vi "HRTF Measurement.vi"(9 "Device Config":T4={"TDT"={"Output"={"Device"=enum."RZ5", "Num"=0}, "Input"=enum."Front Panel"}, "Transducer"="", "Properties"={"Amplifier"=enum."None", "Panic button"=FALSE}, "System"=enum."PXI"}) -> ()   [LabVIEW 2015]
uses:
  EPhys/LV Source/Typedefs/EPhys-Hardware Config.ctl
  PXI DAQ VIs/TDT VIs/Typedefs/TDT-Device Config.ctl
  PXI DAQ VIs/TDT VIs/Typedefs/TDT-Output source.ctl
  PXI DAQ VIs/TDT VIs/Typedefs/TDT-Device ID.ctl
  PXI DAQ VIs/TDT VIs/Typedefs/TDT-Input source.ctl
  EPhys/LV Source/Typedefs/EPhys-Hardware Properties.ctl
  PXI DAQ VIs/Type Defs/Hardware Destination.ctl
  Typedefs/HRTF Config/HRTF Config.xctl
  Utility VIs/Buttons/KCheckmarkBoolean 2.ctl
  Typedefs/HRTF-Result.ctl
  Typedefs/HRTF-Parameters.ctl
  Typedefs/HRTF-Waveform.ctl
  Typedefs/HRTF-Window.ctl
  Typedefs/HRTF-Window Type.ctl
  Typedefs/HRTF-State.ctl
  Typedefs/HRTF-Options.ctl
  Typedefs/HRTF-Hardware Config (TDT).ctl
  Typedefs/HRTF-State Machine Action.ctl
  Typedefs/HRTF-Runtime Data.ctl
  <vilib>/Analysis/2dsp.llb/Real FFT.vi
  <vilib>/Utility/miscctls.llb/LVBoundsTypeDef.ctl
  <vilib>/Analysis/NI_AALPro.lvlib
panel:
  in  "Compute":bool
  in  "Window":T1={"Window"=0, "Length (ms)"=50.0, "Center (ms)"=50.0} {"Window" items=["None", "Rectangle", "Hanning"]}
  in  "Cancel":bool
  in  "Apply":bool
  out "Result":T2
  out "StimDur":dbl format="%#_3g ms"
  in  "wftab":enum32{"Page 1", "Page 2"}(tab)
  in  "Freq Step (Hz)":dbl=50.0
  in  "Seed":i32=50
  in  "Order":i32=50
  in  "Attenuation (dB)":dbl=30.0
  in  "Sample Rate (Hz)":dbl=100000.0
  in  "Waveform":enum16{"Chirp", "MLS"}(ring)
  out "Progress":u8(slide) scale=0.0..1.0
  in  "Elevation":u16(ring) items=["0°", "7.5°", "15°", "22.5°", "30°", "37.5°", "45°", "52.5°", "60°", "67.5°", "75°", "82.5°", "90°", "97.5°", "105°", "112.5°", "120°", "127.5°", "135°", "142.5°", "150°", "157.5°", "165°", "172.5°", "180°"]
  in  "Speaker only":T3
  in  "Start":bool
  in  "Stop":bool
  in  "Subject ID":string
  in  "Config":i32(xcontrol)
  in  "Averages":i32=128
  in  "Data Tab":enum32{"Stimulus", "Response", "HRTFs"}(tab)
  out "StimPhase":cluster{i32, "dx":dbl, "Y":dbl[]}(graph)
  out "StimMag":cluster{i32, "dx":dbl, "Y":dbl[]}(graph)
  out "StimAutocorr":cluster{dbl, "dx":dbl, "Y":dbl[]}(graph) caption="Autocorrelation"
  out "Stimulus (time)":cluster{i32, "dx":dbl, "Y":dbl[]}(graph) caption="Amplitude"
  out "RespTime":cluster{"offset":dbl, "dx":dbl, "Y":dbl[][]}(graph) caption="Amplitude"
  in  "RespFiles":u16(ring) items=["", "Speaker-elev0-az-90", "Speaker-elev0-az-82.5", "Speaker-elev0-az-75", "Speaker-elev0-az-67.5", "Speaker-elev0-az-60", "Speaker-elev0-az-52.5", "Speaker-elev0-az-45"]
  out "RespCorr":cluster{"offset":dbl, "dx":dbl, "Y":dbl[][]}(graph) caption="Impulse Response"
  out "RespMag":cluster{"offset":dbl, "dx":dbl, "Y":dbl[][]}(graph)
  out "RespPhase":cluster{"offset":dbl, "dx":dbl, "Y":dbl[][]}(graph)
  out "Status":string
  in  "HRTFFiles":u16(ring) items=["", "HRTF-elev0-az-90", "HRTF-elev0-az-82.5", "HRTF-elev0-az-75", "HRTF-elev0-az-67.5", "HRTF-elev0-az-60", "HRTF-elev0-az-52.5", "HRTF-elev0-az-45", "HRTF-elev0-az-37.5", "HRTF-elev0-az-30", "HRTF-elev0-az-22.5", "HRTF-elev0-az-15", "HRTF-elev0-az-7.5", "HRTF-elev0-az0", "HRTF-elev0-az7.5", "HRTF-elev0-az15", "HRTF-elev0-az22.5", "HRTF-elev0-az30", "HRTF-elev0-az37.5", "HRTF-elev0-az45", "HRTF-elev0-az52.5", "HRTF-elev0-az60", "HRTF-elev0-az67.5", "HRTF-elev0-az75", "HRTF-elev0-az82.5", "HRTF-elev0-az90"]
  out "HRTFMag":cluster{"offset":dbl, "dx":dbl, "Y":dbl[][]}(graph)
  out "HRTFPhase":cluster{"offset":dbl, "dx":dbl, "Y":dbl[][]}(graph)
  out "HRIR":cluster{"offset":dbl, "dx":dbl, "Y":dbl[][]}(graph) caption="Impulse Response"
  # "Stimulus"
  # "HRTF"
  # "Response"
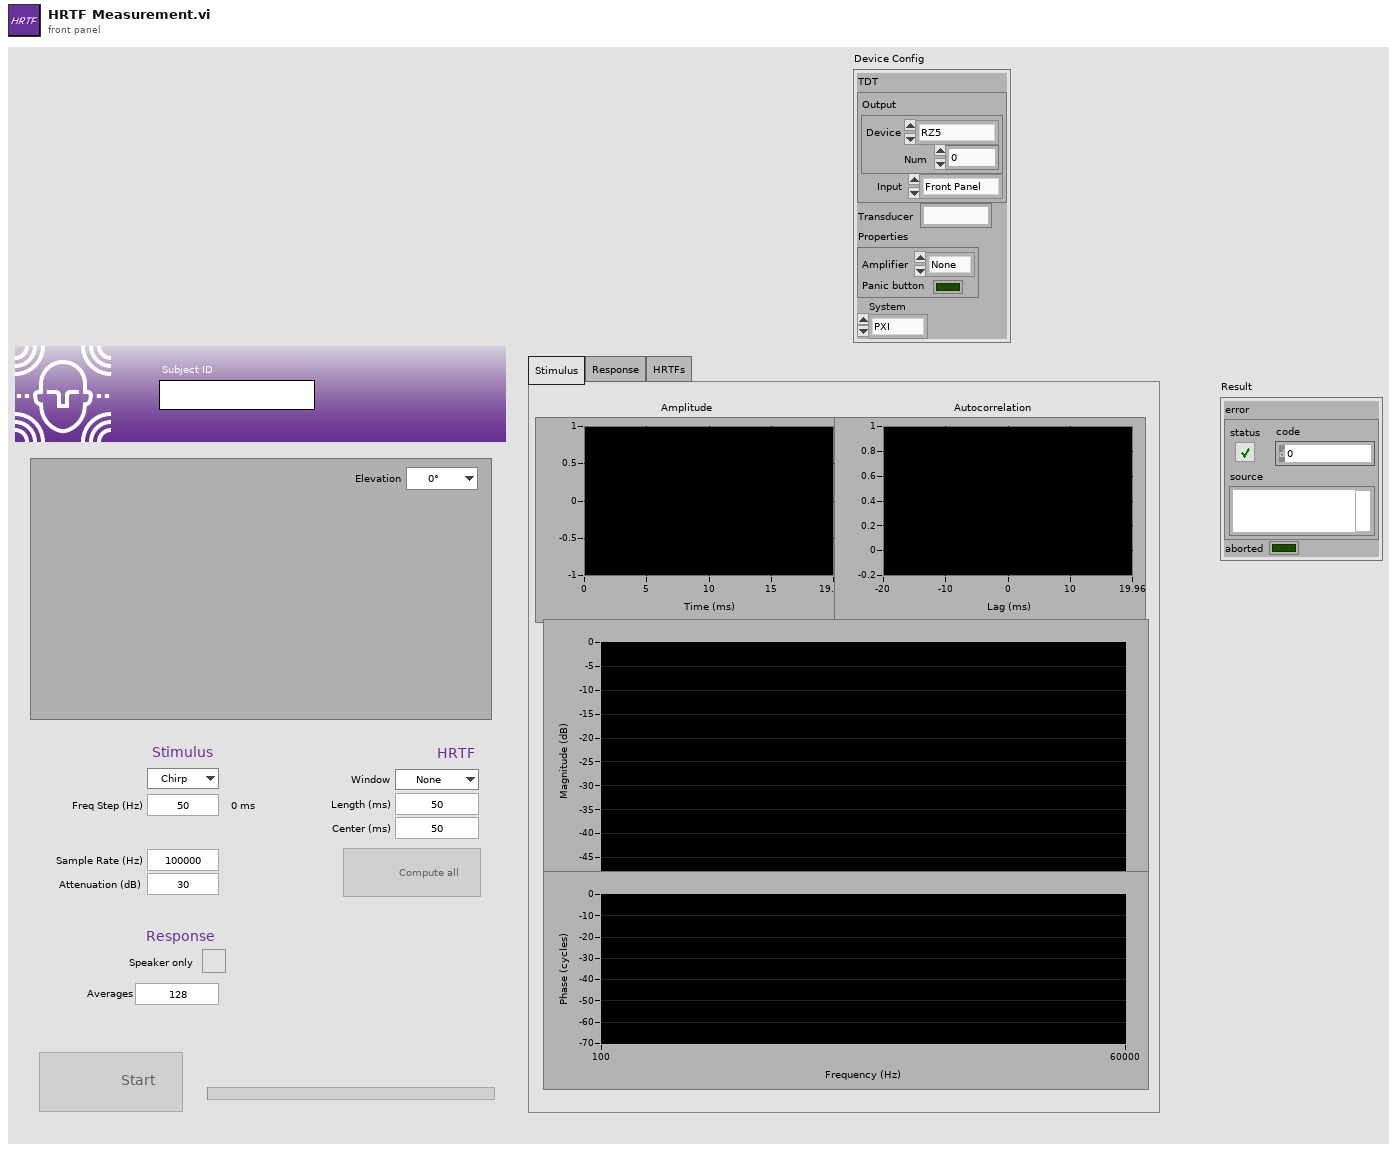
[diagram p1: front panel]
types:
  T1 = cluster{"Window":u16, "Length (ms)":dbl, "Center (ms)":dbl}
  T2 = typedef "HRTF-Result.ctl" = cluster{"error":errorcluster, "aborted":bool}
  T3 = typedef "KCheckmarkBoolean 2.ctl" = bool
  T4 = typedef "EPhys-Hardware Config.ctl" = cluster{"TDT":T5, "Transducer":string, "Properties":T9, "System":T10}
  T5 = typedef "TDT-Device Config.ctl" = cluster{"Output":T6, "Input":T8}
  T6 = typedef "TDT-Output source.ctl" = cluster{"Device":T7, "Num":i32}
  T7 = typedef "TDT-Device ID.ctl" = enum16{"None", "PA5", "RP2", "RL2", "RA16", "RV8", "RX5", "RX6", "RX7", "RX8", "RZ2", "RZ5", "RZ6"}
  T8 = typedef "TDT-Input source.ctl" = enum16{"Front Panel", "RA4LI", "RA16LI"}
  T9 = typedef "EPhys-Hardware Properties.ctl" = cluster{"Amplifier":enum16{"None", "Biosemi", "Eclipse", "Eclipse (N.C.)", "Grass"}, "Panic button":bool}
  T10 = typedef "Hardware Destination.ctl" = enum16{"None", "PXI", "TDT", "NI", "TDTSIM"}
  T11 = typedef "HRTF-Parameters.ctl" = cluster{"Fs (Hz)":dbl, "atten (dB)":dbl, "Waveform":T12, "Freq Res (Hz)":dbl, "Order":i32, "Averages":i32, "seed":i64, "Window":T13}
  T12 = typedef "HRTF-Waveform.ctl" = enum16{"Chirp", "MLS"}
  T13 = typedef "HRTF-Window.ctl" = cluster{"Type":T14, "Length (ms)":dbl, "Center (ms)":dbl}
  T14 = typedef "HRTF-Window Type.ctl" = enum16{"None", "Rectangle", "Hanning"}
  T15 = typedef "HRTF-Options.ctl" = cluster{"Root folder":path, "Elevations":string, "Wait (s)":dbl, "Azimuths":dbl[]}
  T16 = typedef "HRTF-State.ctl" = cluster{"Folder":path, "Elevation":dbl, "iAzimuth":i32, "Mic":i32, "speaker only":bool, "ID":string, "Azimuth":dbl}
  T17 = typedef "LVBoundsTypeDef.ctl" = cluster{"Width":u32, "Height":u32}
  T18 = cluster{"Options":T15, "Params":T11, "State":T16}
  T19 = enum8{"Enabled", "Disabled", "Disabled and Grayed Out"}
  T20 = enum32{"Invalid", "Standard", "Closed", "Hidden", "Minimized", "Maximized"}
  T21 = typedef "LVRangeTypeDef.ctl" = cluster{"Minimum":dbl, "Maximum":dbl, "Increment":dbl, "Minor Increment":dbl, "Start":dbl}
  T22 = typedef "HRTF-Hardware Config (TDT).ctl" = cluster{"Output":T6, "Speaker":cluster{"Channel":i32, "Primary mux":i32, "Secondary mux":i32}, "Right mic":i32, "Left mic":i32}
  T23 = typedef "HRTF-Runtime Data.ctl" = cluster{"StimSpec":cdb[][], "Mic Sum":dbl[][], "df (Hz)":dbl, "dt (ms)":dbl, "Navg":i32, "Nacq":i32, "pts/rep":i32, "reps/frame":i32, "Stimulus":dbl[]}
  T24 = typedef "HRTF-State Machine Action.ctl" = enum16{"Wait", "Init", "Multiplex", "Measure", "Save", "End"}
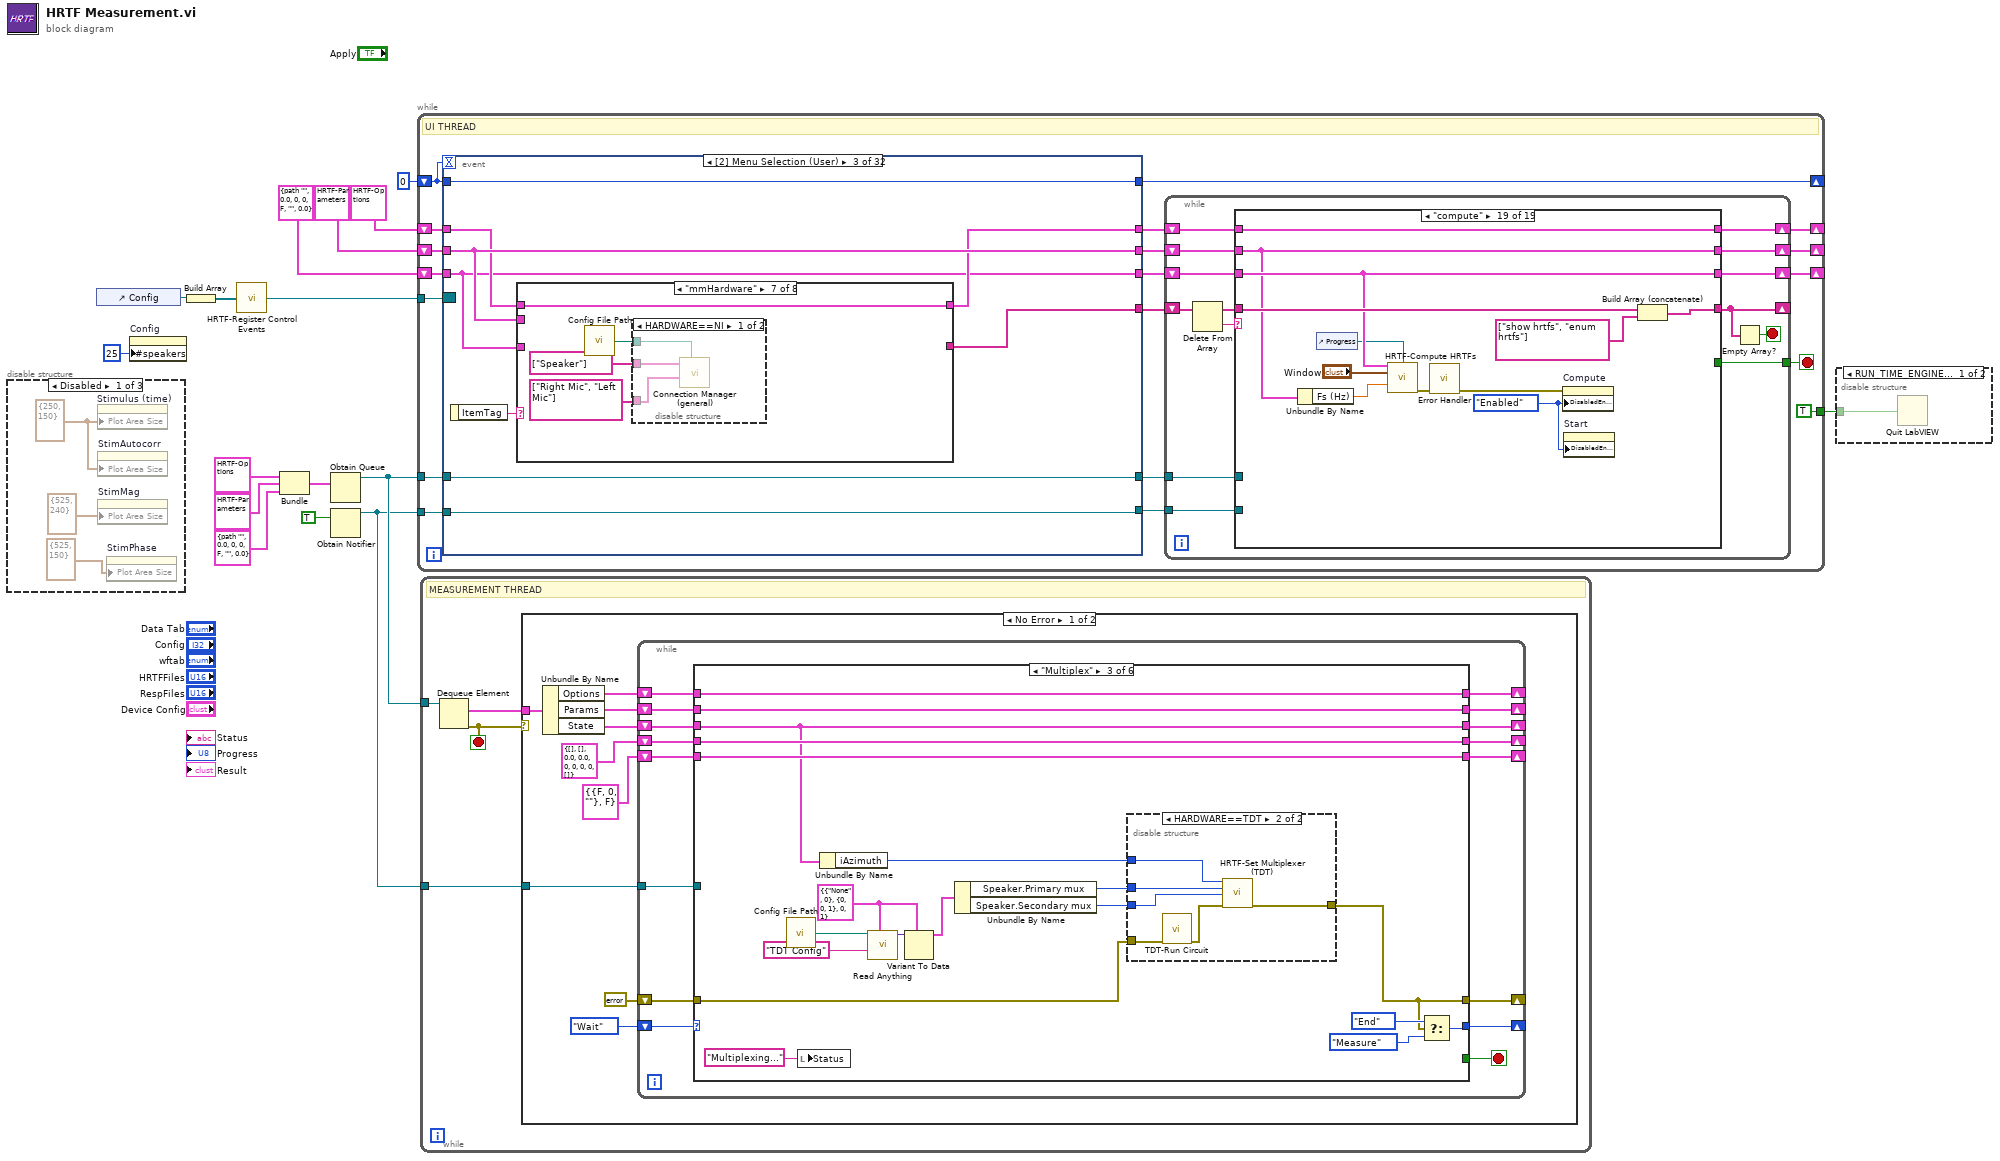
[diagram p0: block diagram]
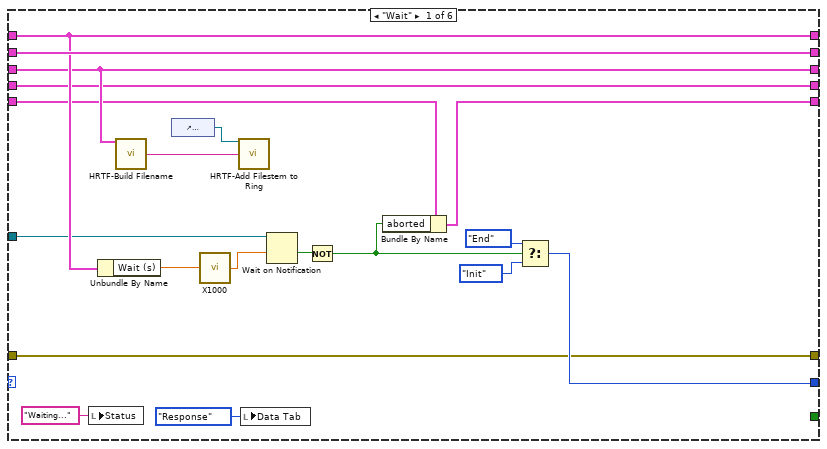
[diagram p2: hidden frame]
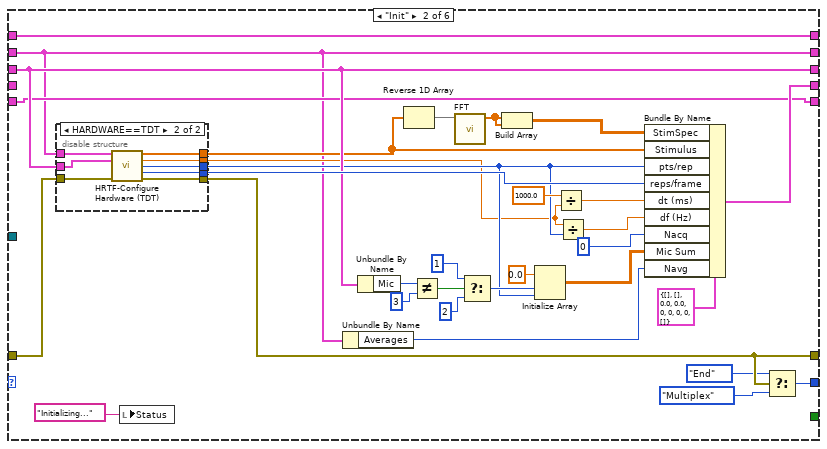
[diagram p3: hidden frame]
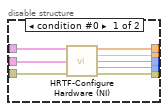
[diagram p4: hidden frame]
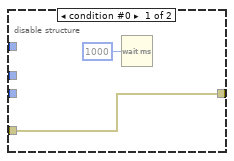
[diagram p5: hidden frame]
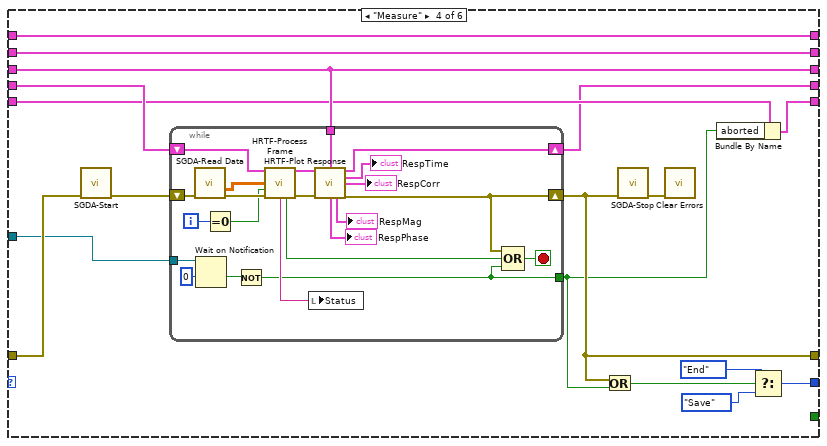
[diagram p6: hidden frame]
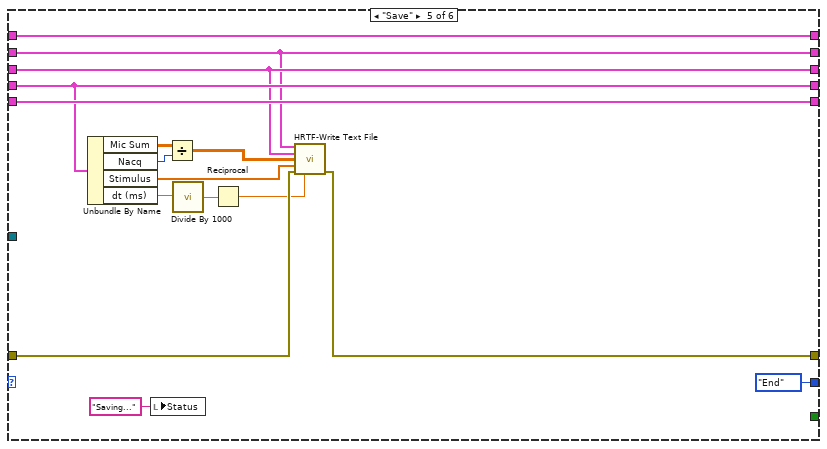
[diagram p7: hidden frame]
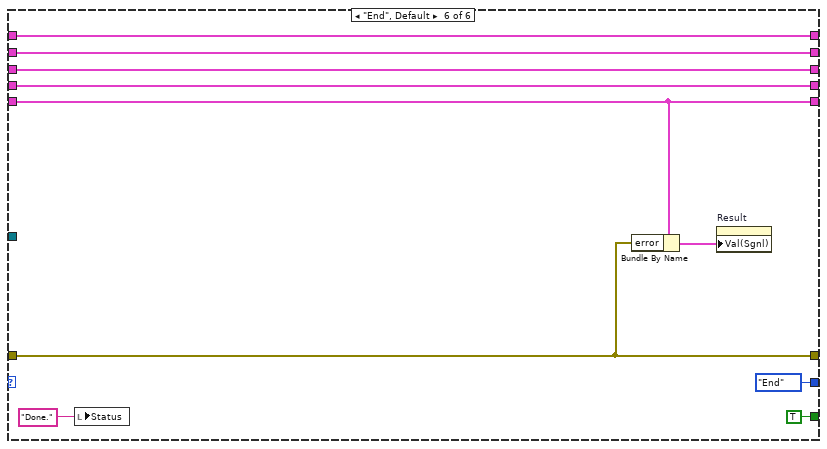
[diagram p8: hidden frame]
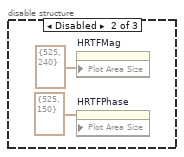
[diagram p10: hidden frame]
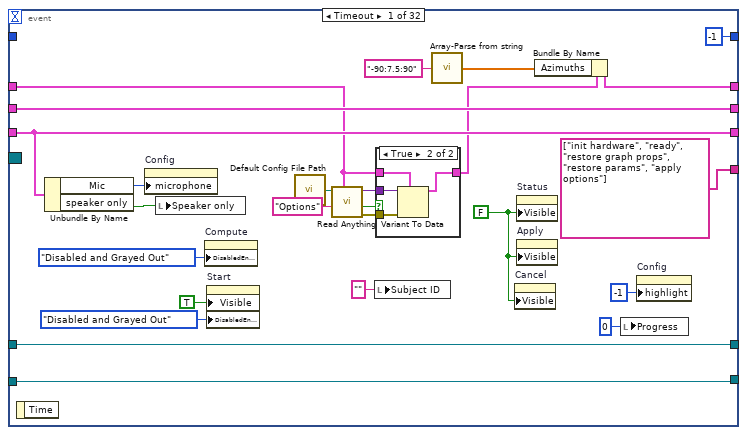
[diagram p12: hidden frame]
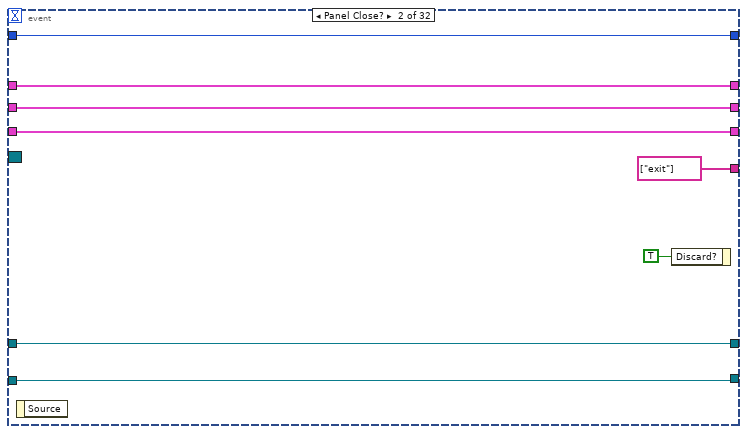
[diagram p14: hidden frame]
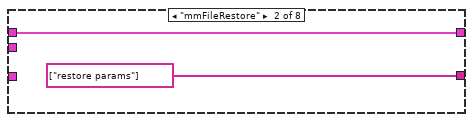
[diagram p16: hidden frame]
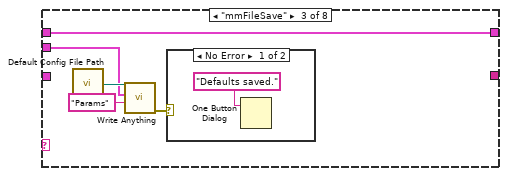
[diagram p17: hidden frame]
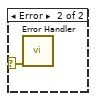
[diagram p18: hidden frame]
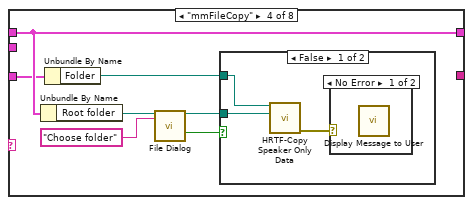
[diagram p19: hidden frame]
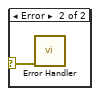
[diagram p20: hidden frame]
diagram:
  n1 = disable-structure shown="Disabled" {
    frame Disabled {
      w19 = T17 {"Width"=250, "Height"=150} ("Plot Area:Size")
      n2 = property on="Stimulus (time)" class="WFGraph (strict)"("Plot Area Size"=w19) -> ()  [unwired: 2 in, 2 out]
      n3 = property on="StimAutocorr" class="WFGraph (strict)"("Plot Area Size"=w19) -> ()  [unwired: 2 in, 2 out]
      n4 = property on="StimMag" class="WFGraph (strict)"("Plot Area Size"=T17 {"Width"=525, "Height"=240} ("Plot Area:Size")) -> ()  [unwired: 2 in, 2 out]
      n5 = property on="StimPhase" class="WFGraph (strict)"("Plot Area Size"=T17 {"Width"=525, "Height"=150} ("Plot Area:Size")) -> ()  [unwired: 2 in, 2 out]
    }
    frame Disabled {
      n6 = property on="HRTFMag" class="WFGraph (strict)"("Plot Area Size"=T17 {"Width"=525, "Height"=240} ("Plot Area:Size")) -> ()  [unwired: 2 in, 2 out]
      n7 = property on="HRTFPhase" class="WFGraph (strict)"("Plot Area Size"=T17 {"Width"=525, "Height"=150} ("Plot Area:Size")) -> ()  [unwired: 2 in, 2 out]
    }
    frame Enabled {
    }
  }
  n8 = control-ref of="Config"() -> (w11:refnum<vi>)
  n9 = property on="Config" class="HRTF Config (strict)"("#speakers"=25) -> ()  [unwired: 2 in, 2 out]
  n10 = Build Array(w11) -> (w10:refnum<vi>[])
  n11 = call "HRTF-Register Control Events.vi"("Refs"=w10) -> ("event registration refnum"=w9:refnum<event-registration>)  [unwired: 13 in, 1 out]
  n12 = Bundle("Options"=T15 {"Root folder"=path "C:/Data", "Elevations"="0:7.5:180", "Wait (s)"=2.0, "Azimuths"=[]}, "Params"=T11 {"Fs (Hz)"=100000.0, "atten (dB)"=20.0, "Waveform"=enum."Chirp", "Freq Res (Hz)"=50.0, "Order"=10, "Averages"=100, "seed"=-1, "Window"={"Type"=enum."None", "Length (ms)"=0.0, "Center (ms)"=0.0}}, "State"=T16 {"Folder"=path "", "Elevation"=0.0, "iAzimuth"=0, "Mic"=0, "speaker only"=FALSE, "ID"="", "Azimuth"=0.0}) -> (w1:T18)  [unwired: 1 in]
  n13 = Obtain Queue(element data type=w1) -> (queue out=w16:refnum<queue>)  [unwired: 4 in, 2 out]
  n14 = Obtain Notifier(notification data type=TRUE) -> (notifier out=w13:refnum<notifier>)  [unwired: 3 in, 2 out]
  n15 = while {
    tunnel: w16 -> [w40]
    shift-right: [w39] -> _
    shift-left: 0 -> [w38]
    shift-right: [w27] -> _
    shift-left: T11 {"Fs (Hz)"=100000.0, "atten (dB)"=20.0, "Waveform"=enum."Chirp", "Freq Res (Hz)"=50.0, "Order"=10, "Averages"=100, "seed"=-1, "Window"={"Type"=enum."None", "Length (ms)"=5.0, "Center (ms)"=2.5}} ("Params") -> [w37]
    tunnel: w13 -> [w36]
    tunnel: w9 -> [w35]
    shift-right: [w26] -> _
    shift-left: T15 {"Root folder"=path "C:/Data", "Elevations"="0:7.5:180", "Wait (s)"=2.0, "Azimuths"=[]} ("Options") -> [w34]
    shift-right: [w28] -> _
    shift-left: T16 {"Folder"=path "", "Elevation"=0.0, "iAzimuth"=0, "Mic"=0, "speaker only"=FALSE, "ID"="", "Azimuth"=0.0} ("State") -> [w33]
    tunnel: [TRUE] -> w5
    stop <- w25 stop-if-true
    # "UI THREAD"
    n16 = event shown="[2] Menu Selection (User)" {
      selector: w35 -> [_ _ _ _ _ _ _ _ _ _ _ _ _ _ _ _ _ _ _ _ _ _ _ _ _ _ _ _ _ _ _ _]
      dyn-events: _ -> [_ _ _ _ _ _ _ _ _ _ _ _ _ _ _ _ _ _ _ _ _ _ _ _ _ _ _ _ _ _ _ _]
      timeout: w38 -> [_ _ _ _ _ _ _ _ _ _ _ _ _ _ _ _ _ _ _ _ _ _ _ _ _ _ _ _ _ _ _ _]
      tunnel: w40 -> [w58 w72 w83 w132 w151 w161 w167 w177 w189 w197 w206 w215 w224 w233 w241 w251 w257 w268 w276 w284 w302 w303 w313 w332 w343 w354 w362 w369 w382 w402 w417 w425]
      tunnel: [-1 w78 w86 w136 w153 w164 w173 w180 w192 w202 w211 w220 w229 w238 w246 w255 w263 w272 w280 w288 w301 w309 w318 w336 w347 w358 w366 w373 w386 w406 w421 w429] -> w39
      tunnel: w38 -> [_ w78 w86 w136 w153 w164 w173 w180 w192 w202 w211 w220 w229 w238 w246 w255 w263 w272 w280 w288 w301 w309 w318 w336 w347 w358 w366 w373 w386 w406 w421 w429]
      tunnel: w37 -> [w61 w77 w85 w135 w152 w163 w168 w179 w191 w199 w208 w217 w226 w235 w243 w254 w259 w271 w279 w287 w300 w308 w317 w335 w346 w357 w365 w372 w385 w405 w420 w428]
      tunnel: [w61 w77 w85 w135 w152 w163 w168 w179 w191 w198 w207 w216 w225 w234 w242 w254 w258 w266 w274 w282 w300 w308 w317 w335 w346 w357 w365 w372 w385 w405 w420 w428] -> w30
      tunnel: w36 -> [w57 w71 w82 w131 w150 w160 w166 w176 w188 w196 w205 w214 w223 w232 w240 w250 w256 w267 w275 w283 w299 w307 w312 w331 w342 w353 w361 w368 w381 w401 w416 w424]
      tunnel: w34 -> [w52 w74 w81 w134 w140 w162 w172 w178 w187 w201 w210 w219 w228 w237 w245 w253 w261 w270 w278 w286 w297 w304 w314 w334 w345 w356 w364 w371 w384 w404 w419 w427]
      tunnel: w33 -> [w59 w75 w79 w133 w147 w158 w170 w175 w190 w200 w209 w218 w227 w236 w244 w252 w260 w269 w277 w285 w298 w305 w315 w333 w344 w355 w363 w370 w383 w403 w418 w426]
      tunnel: [w44 w74 w80 w134 w140 w162 w172 w178 w187 w201 w210 w219 w228 w237 w245 w253 w261 w270 w278 w286 w297 w304 w314 w334 w345 w356 w364 w371 w384 w404 w419 w427] -> w31
      tunnel: [w59 w75 w79 w133 w148 w158 w169 w175 w183 w200 w209 w218 w227 w236 w244 w249 w260 w269 w277 w285 w298 w305 w315 w333 w344 w355 w363 w370 w383 w403 w418 w426] -> w29
      tunnel: [string[] ["init hardware", "ready", "restore graph props", "restore params", "apply options"] string[] ["exit"] w84 _ string[] ["show hrtfs", "enum hrtfs", "enum work", "enable start"] ("String") _ string[] ["enable start"] ("String") string[] ["enable start"] ("String") string[] ["show hrtfs", "enum hrtfs", "enum work"] ("String") string[] ["plot stim"] ("String") string[] ["plot stim"] ("String") string[] ["plot stim"] ("String") string[] ["plot stim"] ("String") string[] ["plot stim"] ("String") _ string[] ["enum work"] ("String") _ string[] ["update window"] ("String") _ _ string[] ["do next"] ("String") _ w311 _ _ _ string[] ["read work"] ("String") string[] ["read hrtf"] ("String") w375 w395 _ string[] ["compute"] ("String")] -> w32
      tunnel: [w58 w72 w83 w132 w151 w161 w167 w177 w189 w197 w206 w215 w224 w233 w241 w251 w257 w268 w276 w284 w302 w303 w313 w332 w343 w354 w362 w369 w382 w402 w417 w425] -> w24
      tunnel: [w57 w71 w82 w131 w150 w160 w166 w176 w188 w196 w205 w214 w223 w232 w240 w250 w256 w267 w275 w283 w295 w307 w312 w331 w342 w353 w361 w368 w381 w401 w416 w424] -> w23
      event Timeout {
        w48 = FALSE ("Visible")
        n17 = event-data() -> ()  [unwired: 1 in, 1 out]
        n18 = Unbundle By Name(w59) -> ("Mic"=w60:i32, "speaker only"=w49:bool)
        n19 = property on="Config" class="HRTF Config (strict)"("microphone"=w60) -> ()  [unwired: 2 in, 2 out]
        n20 = local write "Speaker only"(w49) -> ()
        n21 = property on="Compute" class="Bool"("DisabledEnum"=T19."Disabled and Grayed Out" ("Disabled")) -> ()  [unwired: 2 in, 2 out]
        n22 = property on="Start" class="Bool"("Visible"=TRUE, "DisabledEnum"=T19."Disabled and Grayed Out" ("Disabled")) -> ()  [unwired: 2 in, 2 out]
        n23 = call "Default Config File Path.vi"() -> ("Default config file name"=w55:path)
        n24 = call "Read Anything.vi"("Type of Anything"=w52, "Section Name (Name of \"Type of Anything\")"="Options" ("Section Name (Name of \"Type of Anything\")"), "Path (dialog)"=w55) -> ("Error Out"=w56:errorcluster, "Found?"=w54:bool, "Anything"=w53:variant)  [unwired: 6 in]
        n25 = local write "Subject ID"("" ("Subject ID")) -> ()
        n26 = case shown="True" w54 {
          tunnel: w56 -> [_ w70]
          tunnel: w53 -> [_ w69]
          tunnel: w52 -> [w66 w68]
          tunnel: [w66 w67] -> w51
          frame False {
          }
          frame True {
            n27 = Variant To Data(error in=w70, type=w68, Variant=w69) -> (data=w67:T15)  [unwired: 1 out]
          }
        }
        n28 = call "Array-Parse from string.vi"("String"="-90:7.5:90") -> ("Array"=w43:dbl[])  [unwired: 13 in, 1 out]
        n29 = property on="Cancel" class="Bool"("Visible"=w48) -> ()  [unwired: 2 in, 2 out]
        n30 = property on="Status" class="Str"("Visible"=w48) -> ()  [unwired: 2 in, 2 out]
        n31 = property on="Apply" class="Bool"("Visible"=w48) -> ()  [unwired: 2 in, 2 out]
        n32 = Bundle By Name(cluster=w51, "Azimuths"=w43) -> (w44:T15)
        n33 = local write "Progress"(u8 0 ("Progress")) -> ()
        n34 = property on="Config" class="HRTF Config (strict)"("highlight"=-1) -> ()  [unwired: 2 in, 2 out]
      }
      event Panel Close? {
        n35 = event-data() -> ()  [unwired: 1 in, 1 out]
        n36 = event-data("Discard?"=TRUE) -> ()  [unwired: 1 in, 1 out]
      }
      event Menu Selection (User) {
        n37 = event-data() -> ("ItemTag"=w87:string)  [unwired: 1 in]
        n38 = case shown="\"mmHardware\"" w87 {
          tunnel: w85 -> [_ _ w93 _ _ _ _ _]
          tunnel: [_ string[] ["restore params"] _ _ string[] ["exit"] w111 _ _] -> w84
          tunnel: w81 -> [w88 w89 w91 w104 w109 w114 w122 w127]
          tunnel: [w88 w89 w91 w104 w109 w112 w122 w127] -> w80
          tunnel: w79 -> [_ _ _ w99 _ _ _ _]
          frame "False", Default {
          }
          frame "mmFileRestore" {
          }
          frame "mmFileSave" {
            n39 = call "Default Config File Path.vi"() -> ("Default config file name"=w95:path)
            n40 = call "Write Anything.vi"("Section Name (Name of \"Anything\")"="Params" ("Section Name (Name of \"Anything\")"), "Anything"=w93, "Path (dialog)"=w95) -> ("Error Out"=w92:errorcluster)  [unwired: 7 in, 1 out]
            n41 = case shown="No Error" w92 {
              selector: w92 -> [_ w97]
              frame No Error {
                n42 = One Button Dialog(message="Defaults saved.") -> ()  [unwired: 1 in, 1 out]
              }
              frame Error {
                n43 = call "Error Handler.vi"("error in (no error)"=w97) -> ()  [unwired: 13 in, 2 out]
              }
            }
          }
          frame "mmFileCopy" {
            n44 = Unbundle By Name(w104) -> ("Root folder"=w103:path)
            n45 = Unbundle By Name(w99) -> ("Folder"=w98:path)
            n46 = call "File Dialog"("start path"=w103, "prompt"="Choose folder") -> ("selected path"=w100:path, "cancelled"=w101:bool)  [unwired: 10 in, 2 out]
            n47 = case shown="False" w101 {
              tunnel: w100 -> [w107 _]
              tunnel: w98 -> [w106 _]
              frame False {
                n48 = call "HRTF-Copy Speaker Only Data.vi"("to"=w106, "from"=w107) -> ("error out"=w105:errorcluster)  [unwired: 13 in]
                n49 = case shown="No Error" w105 {
                  selector: w105 -> [_ w108]
                  frame No Error {
                    n50 = call "Display Message to User"() -> ()  [unwired: 10 in, 2 out]
                  }
                  frame Error {
                    n51 = call "Error Handler.vi"("error in (no error)"=w108) -> ()  [unwired: 13 in, 2 out]
                  }
                }
              }
              frame True {
              }
            }
          }
          frame "mmFileExit" {
          }
          frame "mmOptions" {
            n52 = call "HRTF-Options Dialog.vi"("Options in"=w114) -> ("Options out"=w112:T15, "Canceled?"=w113:bool)  [unwired: 13 in]
            n53 = case shown="False" w113 {
              tunnel: w112 -> [w116 _]
              tunnel: [string[] ["apply options"] ("String") _] -> w111
              frame False {
                n54 = call "Default Config File Path.vi"() -> ("Default config file name"=w118:path)
                n55 = call "Write Anything.vi"("Section Name (Name of \"Anything\")"="Options" ("Section Name (Name of \"Anything\")"), "Anything"=w116, "Path (dialog)"=w118) -> ()  [unwired: 7 in, 2 out]
              }
              frame True {
              }
            }
          }
          frame "mmHardware" {
            n56 = call "Config File Path.vi"() -> ("Default config file name"=w119:path)  [unwired: 1 in]
            n57 = disable-structure shown="HARDWARE==NI" {
              disable-tunnel: string[] ["Speaker"] ("Custom Outputs") -> [w125 _]
              disable-tunnel: string[] ["Right Mic", "Left Mic"] ("Custom Outputs") -> [w124 _]
              disable-tunnel: w119 -> [w123 w126]
              frame condition #0 {
                n58 = call "Connection Manager (general).vi"("Path"=w123, "Custom Inputs"=w124, "Custom Outputs"=w125) -> ()  [unwired: 8 in, 1 out]
              }
              frame condition #1 (active) {
                n59 = call "HRTF-Devices Dialog (TDT).vi"("Path"=w126) -> ()  [unwired: 14 in, 1 out]
              }
            }
          }
          frame "mmHelpAbout" {
            n60 = call "HRTF-About Box.vi"() -> ()  [unwired: 12 in]
          }
        }
      }
      event "Subject ID": Value Change {
        n61 = event-data() -> ("NewVal"=w128:string)  [unwired: 1 in]
        n62 = Empty String/Path?(string/path=w128) -> (empty?=w130:bool)
        n63 = Not(x=w130) -> (.not. x?=w129:bool)
        n64 = property on="Apply" class="Bool"("Visible"=w129) -> ()  [unwired: 2 in, 2 out]
        n65 = property on="Cancel" class="Bool"("Visible"=w129) -> ()  [unwired: 2 in, 2 out]
      }
      event "Apply": Value Change {
        w139 = cluster{"offset":dbl, "dx":dbl, "Y":dbl[][]} {"offset"=0.0, "dx"=0.0, "Y"=[]} ("RespTime")
        w149 = FALSE ("Visible")
        n66 = event-data() -> ()  [unwired: 1 in, 1 out]
        n67 = Unbundle By Name(w140) -> ("Root folder"=w146:path)
        n68 = property on="Apply" class="Bool"("Visible"=w149) -> ()  [unwired: 2 in, 2 out]
        n69 = property on="Cancel" class="Bool"("Visible"=w149) -> ()  [unwired: 2 in, 2 out]
        n70 = Build Path(base path=w146, name or relative path="Subject ID") -> (appended path=w143:path)
        n71 = local write "RespTime"(w139) -> ()
        n72 = local write "RespCorr"(w139) -> ()
        n73 = local write "RespMag"(w139) -> ()
        n74 = local write "RespPhase"(w139) -> ()
        n75 = call "FileIO-File or Folder Exists.vi"("path"=w143) -> ("Exists?"=w142:bool, "dup path"=w141:path)  [unwired: 7 in, 2 out]
        n76 = case shown="False" w142 {
          tunnel: w141 -> [w156 _]
          frame False {
            n77 = Create Folder(path (use dialog)=w156) -> ()  [unwired: 2 in, 3 out]
            n78 = Build Path(base path=w156, name or relative path="work") -> (appended path=w155:path)
            n79 = Create Folder(path (use dialog)=w155) -> ()  [unwired: 2 in, 3 out]
          }
          frame True {
          }
        }
        n80 = Bundle By Name(cluster=w147, "ID"="Subject ID", "Folder"=w143, "Azimuth"=nan) -> (w148:T16)
        n81 = property on="Compute" class="Bool"("DisabledEnum"=T19."Enabled" ("Disabled")) -> ()  [unwired: 2 in, 2 out]
      }
      event "Cancel": Value Change {
        w159 = FALSE ("Visible")
        n82 = event-data() -> ()  [unwired: 1 in, 1 out]
        n83 = Unbundle By Name(w158) -> ("ID"=w157:string)
        n84 = local write "Subject ID"(w157) -> ()
        n85 = property on="Apply" class="Bool"("Visible"=w159) -> ()  [unwired: 2 in, 2 out]
        n86 = property on="Cancel" class="Bool"("Visible"=w159) -> ()  [unwired: 2 in, 2 out]
      }
      event User Event {
        n87 = event-data() -> ("Value"=w171:i32)  [unwired: 1 in]
        n88 = Bundle By Name(cluster=w170, "Mic"=w171) -> (w169:T16)
      }
      event User Event {
        n89 = event-data() -> ()  [unwired: 1 in, 1 out]
      }
      event "Elevation": Value Change {
        n90 = event-data() -> ()  [unwired: 1 in, 1 out]
        n91 = Unbundle By Name(w187) -> ("Elevations"=w186:string)
        n92 = call "Array-Parse from string.vi"("String"=w186) -> ("Array"=w185:dbl[])  [unwired: 13 in, 1 out]
        n93 = Index Array(array=w185, index="Elevation") -> (element=w182:dbl)
        n94 = Bundle By Name(cluster=w190, "Elevation"=w182) -> (w183:T16)
      }
      event "Waveform": Value Change {
        n95 = event-data() -> ()  [unwired: 1 in, 1 out]
        n96 = Bundle By Name(cluster=w199, "Waveform"="Waveform") -> (w198:T11)
        n97 = To Long Integer(number="Waveform") -> (32bit integer=w194:i32)
        n98 = local write "wftab"(w194) -> ()
      }
      event "Freq Step (Hz)": Value Change {
        n99 = event-data() -> ()  [unwired: 1 in, 1 out]
        n100 = Bundle By Name(cluster=w208, "Freq Res (Hz)"="Freq Step (Hz)") -> (w207:T11)
      }
      event "Order": Value Change {
        n101 = event-data() -> ()  [unwired: 1 in, 1 out]
        n102 = Bundle By Name(cluster=w217, "Order"="Order") -> (w216:T11)
      }
      event "Seed": Value Change {
        n103 = event-data() -> ()  [unwired: 1 in, 1 out]
        n104 = Bundle By Name(cluster=w226, "seed"="Seed") -> (w225:T11)
      }
      event "Sample Rate (Hz)": Value Change {
        n105 = event-data() -> ()  [unwired: 1 in, 1 out]
        n106 = Bundle By Name(cluster=w235, "Fs (Hz)"="Sample Rate (Hz)") -> (w234:T11)
      }
      event "Attenuation (dB)": Value Change {
        n107 = event-data() -> ()  [unwired: 1 in, 1 out]
        n108 = Bundle By Name(cluster=w243, "atten (dB)"="Attenuation (dB)") -> (w242:T11)
      }
      event Value Change {
        n109 = event-data() -> ()  [unwired: 1 in, 1 out]
        n110 = Bundle By Name(cluster=w252, "speaker only"="Speaker only") -> (w249:T16)
      }
      event "Averages": Value Change {
        n111 = event-data() -> ()  [unwired: 1 in, 1 out]
        n112 = Bundle By Name(cluster=w259, "Averages"="Averages") -> (w258:T11)
      }
      event "Window.Window": Value Change {
        n113 = event-data() -> ("NewVal"=w264:u16)  [unwired: 1 in]
        n114 = Bundle By Name(cluster=w271, "Window.Type"=w264) -> (w266:T11)
      }
      event "Window.Length (ms)": Value Change {
        n115 = event-data() -> ("NewVal"=w273:dbl)  [unwired: 1 in]
        n116 = Bundle By Name(cluster=w279, "Window.Length (ms)"=w273) -> (w274:T11)
      }
      event "Window.Center (ms)": Value Change {
        n117 = event-data() -> ("NewVal"=w281:dbl)  [unwired: 1 in]
        n118 = Bundle By Name(cluster=w287, "Window.Center (ms)"=w281) -> (w282:T11)
      }
      event "Start": Value Change {
        n119 = event-data() -> ()  [unwired: 1 in, 1 out]
        n120 = Cancel Notification(0:w299) -> (8:w295:refnum<notifier>)  [unwired: 1 in, 2 out]
        n121 = property on="Config" class="HRTF Config (strict)"() -> ("selection"=w294:i32[])  [unwired: 2 in, 2 out]
        n122 = Array Size(array=w294) -> (size(s)=w293:i32)
        n123 = property on="Progress" class="Slide (strict)"("Scale.Maximum"=w293, "Value"=u8 0 ("Progress")) -> ()  [unwired: 2 in, 2 out]
        n124 = property on="RespFiles" class="Ring (strict)"("DisabledEnum"=T19."Disabled and Grayed Out" ("Disabled")) -> ()  [unwired: 2 in, 2 out]
        n125 = property on="Status" class="Str"("Visible"=TRUE) -> ()  [unwired: 2 in, 2 out]
        n126 = property on="Start" class="Bool"("Visible"=FALSE) -> ()  [unwired: 2 in, 2 out]
      }
      event "Stop": Value Change {
        n127 = event-data() -> ()  [unwired: 1 in, 1 out]
        n128 = Send Notification(notification=TRUE ("element"), notifier=w307) -> ()  [unwired: 1 in, 2 out]
      }
      event Value Change {
        n129 = event-data() -> ("NewVal.error"=w316:errorcluster, "NewVal.aborted"=w310:bool)  [unwired: 1 in]
        n130 = case shown="No Error" w316 {
          selector: w316 -> [_ w326]
          tunnel: [w320 string[] ["end run"] ("String")] -> w311
          tunnel: w310 -> [w319 _]
          frame No Error {
            n131 = case shown="False" w319 {
              tunnel: [w322 string[] ["end run"] ("String")] -> w320
              frame False {
                n132 = Build Array("do next", "update" ("String")) -> (w322:string[])
              }
              frame True {
              }
            }
          }
          frame Error {
            n133 = call "Error Handler.vi"("error in (no error)"=w326) -> ()  [unwired: 13 in, 2 out]
          }
        }
      }
      event "StimPhase": Scale Range Change {
        n134 = event-data() -> ("ScaleRef"=w330:refnum<vi>, "NewRange"=w327:T21)  [unwired: 1 in]
        n135 = property on="StimPhase" class="WFGraph (strict)"() -> ("XScale"=w329:refnum<vi>)  [unwired: 2 in, 2 out]
        n136 = Equal?(x=w329, y=w330) -> (x = y?=w328:bool)
        n137 = case shown="True" w328 {
          tunnel: w327 -> [_ w337]
          frame False {
          }
          frame True {
            n138 = property on="StimMag" class="WFGraph (strict)"("XScale.Range"=w337) -> ()  [unwired: 2 in, 2 out]
          }
        }
      }
      event "RespPhase": Scale Range Change {
        n139 = event-data() -> ("ScaleRef"=w341:refnum<vi>, "NewRange"=w338:T21)  [unwired: 1 in]
        n140 = property on="RespPhase" class="WFGraph (strict)"() -> ("XScale"=w340:refnum<vi>)  [unwired: 2 in, 2 out]
        n141 = Equal?(x=w340, y=w341) -> (x = y?=w339:bool)
        n142 = case shown="True" w339 {
          tunnel: w338 -> [_ w348]
          frame False {
          }
          frame True {
            n143 = property on="RespMag" class="WFGraph (strict)"("XScale.Range"=w348) -> ()  [unwired: 2 in, 2 out]
          }
        }
      }
      event "HRTFPhase": Scale Range Change {
        n144 = event-data() -> ("ScaleRef"=w352:refnum<vi>, "NewRange"=w349:T21)  [unwired: 1 in]
        n145 = property on="HRTFPhase" class="WFGraph (strict)"() -> ("XScale"=w351:refnum<vi>)  [unwired: 2 in, 2 out]
        n146 = Equal?(x=w351, y=w352) -> (x = y?=w350:bool)
        n147 = case shown="True" w350 {
          tunnel: w349 -> [_ w359]
          frame False {
          }
          frame True {
            n148 = property on="HRTFMag" class="WFGraph (strict)"("XScale.Range"=w359) -> ()  [unwired: 2 in, 2 out]
          }
        }
      }
      event "RespFiles": Value Change {
        n149 = event-data() -> ()  [unwired: 1 in, 1 out]
      }
      event "HRTFFiles": Value Change {
        n150 = event-data() -> ()  [unwired: 1 in, 1 out]
      }
      event "HRTFFiles": Mouse Wheel {
        n151 = event-data() -> ("Delta"=w377:i32)  [unwired: 1 in]
        n152 = property on="HRTFFiles" class="Ring (strict)"() -> ("Value"=w378:u16, "Strings []"=w379:string[])  [unwired: 2 in, 2 out]
        n153 = Array Size(array=w379) -> (size(s)=w376:i32)
        n154 = Decrement(x=w376) -> (x-1=w374:i32)
        n155 = Greater Than 0?(x=w374) -> (x > 0?=w380:bool)
        n156 = case shown="True" w380 {
          tunnel: w378 -> [_ w393]
          tunnel: w377 -> [_ w392]
          tunnel: w374 -> [_ w390]
          tunnel: [_ string[] ["read hrtf"] ("String")] -> w375
          frame False {
          }
          frame True {
            n157 = Subtract(x=w393, y=w392) -> (x-y=w391:i32)
            n158 = In Range and Coerce(upper limit=w390, x=w391, lower limit=1) -> (coerced(x)=w388:i32)  [unwired: 1 out]
            n159 = local write "HRTFFiles"(w388) -> ()
          }
        }
      }
      event "RespFiles": Mouse Wheel {
        n160 = event-data() -> ("Delta"=w397:i32)  [unwired: 1 in]
        n161 = property on="RespFiles" class="Ring (strict)"() -> ("Value"=w398:u16, "Strings []"=w399:string[])  [unwired: 2 in, 2 out]
        n162 = Array Size(array=w399) -> (size(s)=w396:i32)
        n163 = Decrement(x=w396) -> (x-1=w394:i32)
        n164 = Greater Than 0?(x=w394) -> (x > 0?=w400:bool)
        n165 = case shown="True" w400 {
          tunnel: w398 -> [_ w413]
          tunnel: w397 -> [_ w412]
          tunnel: w394 -> [_ w410]
          tunnel: [_ string[] ["read work"] ("String")] -> w395
          frame False {
          }
          frame True {
            n166 = Subtract(x=w413, y=w412) -> (x-y=w411:i32)
            n167 = In Range and Coerce(upper limit=w410, x=w411, lower limit=1) -> (coerced(x)=w408:i32)  [unwired: 1 out]
            n168 = local write "RespFiles"(w408) -> ()
          }
        }
      }
      event "HRTFMag": Scale Range Change {
        n169 = event-data() -> ("CtlRef"=w415:refnum<vi>)  [unwired: 1 in]
        n170 = call "Config File Path.vi"() -> ("Default config file name"=w414:path)  [unwired: 1 in]
        n171 = call "Write Graph Properties.vi"("Config File"=w414, "WFGraph Refnum"=w415) -> ()  [unwired: 13 in, 1 out]
      }
      event "Compute": Value Change {
        w422 = T19."Disabled and Grayed Out" ("Disabled")
        n172 = event-data() -> ()  [unwired: 1 in, 1 out]
        n173 = property on="Compute" class="Bool"("DisabledEnum"=w422) -> ()  [unwired: 2 in, 2 out]
        n174 = property on="Start" class="Bool"("DisabledEnum"=w422) -> ()  [unwired: 2 in, 2 out]
      }
    }
    n175 = while {
      shift-right: [w434] -> _
      shift-left: w32 -> [w443]
      shift-right: [w437] -> w26
      shift-left: w31 -> [w440]
      shift-right: [w436] -> w27
      shift-left: w30 -> [w439]
      shift-right: [w435] -> w28
      shift-left: w29 -> [w438]
      tunnel: [w432] -> w25
      tunnel: w24 -> [w431]
      tunnel: w23 -> [w430]
      stop <- w433 stop-if-true
      n176 = Delete From Array(array=w443) -> (deleted portion=w442:string, array with subset deleted=w441:string[])  [unwired: 2 in]
      n177 = case shown="\"compute\"" w442 {
        tunnel: w441 -> [w444 w452 _ w466 w485 w489 w512 w524 w534 _ w561 w571 w581 w591 w605 w625 w636 w650 w663]
        tunnel: w440 -> [w447 w451 w464 w469 w488 w492 w514 w526 w536 w540 w558 w570 w580 w593 w607 w627 w639 w652 w664]
        tunnel: w439 -> [w446 w454 w463 w468 w487 w491 w507 w523 w533 w545 w562 w572 w582 w592 w606 w626 w638 w651 w660]
        tunnel: w438 -> [w445 w453 w462 w467 w486 w490 w513 w525 w535 w544 w559 w568 w578 w587 w604 w623 w637 w644 w662]
        tunnel: [w447 w451 w464 w469 w488 w492 w514 w526 w536 w540 w558 w570 w580 w593 w607 w627 w639 w652 w664] -> w437
        tunnel: [w446 w454 w463 w468 w487 w491 w506 w523 w533 w545 w562 w572 w582 w592 w606 w626 w638 w651 w660] -> w436
        tunnel: [w445 w453 w462 w467 w486 w490 w513 w525 w535 w543 w559 w568 w578 w587 w604 w623 w637 w644 w662] -> w435
        tunnel: [w444 w452 string[] [] w466 w485 w489 w498 w524 w534 w542 w561 w571 w581 w591 w605 w619 w636 w650 w655] -> w434
        tunnel: [_ _ TRUE _ _ _ _ _ _ _ _ _ _ _ _ _ _ _ _] -> w432
        tunnel: w431 -> [_ _ w459 _ _ _ _ _ _ w546 _ _ _ _ _ _ _ _ _]
        tunnel: w430 -> [_ _ w458 _ _ _ _ _ _ _ _ _ _ _ _ _ _ _ _]
        frame "False", Default {
        }
        frame "apply options" {
          n178 = Unbundle By Name(w451) -> ("Elevations"=w450:string)
          n179 = call "Array-Parse from string.vi"("String"=w450) -> ("Array"=w449:dbl[])  [unwired: 13 in, 1 out]
          n180 = for {
            tunnel: w449 -> [w457] mode=indexing
            tunnel: [w455] -> w448 mode=indexing
            n181 = Format Into String(format string="%#g°", w457) -> (resulting string=w455:string)  [unwired: 2 in, 1 out]
          }
          n182 = property on="Elevation" class="Ring (strict)"("Strings []"=w448) -> ()  [unwired: 2 in, 2 out]
        }
        frame "exit" {
          n183 = Release Queue(queue=w459) -> ()  [unwired: 2 in, 3 out]
          n184 = Release Notifier(notifier=w458) -> ()  [unwired: 2 in, 3 out]
          n185 = disable-structure shown="HARDWARE==TDT" {
            disable-tunnel: [_ w465] -> _
            frame condition #0 {
              n186 = call "Abort notifier.vi"() -> ()  [unwired: 6 in, 2 out]
            }
            frame condition #1 (active) {
              n187 = call "TDT-Close ActiveX.vi"() -> ("error out"=w465:errorcluster)  [unwired: 15 in]
            }
          }
        }
        frame "init hardware" {
          n188 = disable-structure shown="HARDWARE==TDT" {
            frame condition #0 {
              n189 = vi-ref "PXI DAQ Server.vi"() -> (w471:refnum<vi>)
              n190 = call "Spawn VI.vi"("State"=T20."Hidden", "VI reference"=w471) -> ()  [unwired: 8 in, 2 out]
            }
            frame condition #1 (active) {
              w475 = T22 {"Output"={"Device"=enum."None", "Num"=0}, "Speaker"={"Channel"=0, "Primary mux"=0, "Secondary mux"=1}, "Right mic"=0, "Left mic"=1} ("TDT")
              n191 = call "Config File Path.vi"() -> ("Default config file name"=w476:path)  [unwired: 1 in]
              n192 = call "Read Anything.vi"("Type of Anything"=w475, "Section Name (Name of \"Type of Anything\")"="TDT Config" ("Section Name (Name of \"Type of Anything\")"), "Path (dialog)"=w476) -> ("Error Out"=w479:errorcluster, "Anything"=w478:variant)  [unwired: 6 in, 1 out]
              n193 = Variant To Data(error in=w479, type=w475, Variant=w478) -> (data=w480:T22, error out=w481:errorcluster)
              n194 = Unbundle By Name(w480) -> ("Output"=w472:T6)
              n195 = Bundle By Name(cluster=T5 {"Output"={"Device"=enum."None", "Num"=0}, "Input"=enum."Front Panel"} ("TDT-Device Config"), "Output"=w472) -> (w473:T5)
              n196 = call "TDT-Init ActiveX.vi"("TDT-Device Config"=w473, "error in (no error)"=w481) -> ("error out"=w482:errorcluster)  [unwired: 10 in, 3 out]
              n197 = call "Error Handler.vi"("error in (no error)"=w482) -> ()  [unwired: 13 in, 2 out]
            }
          }
        }
        frame "restore graph props" {
          n198 = control-ref of="HRTFMag"() -> (w483:refnum<vi>)
          n199 = call "Default Config File Path.vi"() -> ("Default config file name"=w484:path)
          n200 = call "Read Graph Properties.vi"("Config File"=w484, "WFGraph Refnum"=w483) -> ()  [unwired: 12 in, 2 out]
        }
        frame "ready" {
          n201 = call "RunExe-Send Target Ready.vi"() -> ()  [unwired: 15 in, 1 out]
        }
        frame "restore params" {
          n202 = call "Default Config File Path.vi"() -> ("Default config file name"=w510:path)
          n203 = call "Read Anything.vi"("Type of Anything"=w507, "Section Name (Name of \"Type of Anything\")"="Params" ("Section Name (Name of \"Type of Anything\")"), "Path (dialog)"=w510) -> ("Error Out"=w511:errorcluster, "Found?"=w509:bool, "Anything"=w508:variant)  [unwired: 6 in]
          n204 = case shown="True" w509 {
            tunnel: w511 -> [_ w519]
            tunnel: w508 -> [_ w518]
            tunnel: w507 -> [w515 w517]
            tunnel: [w515 w516] -> w506
            frame False {
            }
            frame True {
              n205 = Variant To Data(error in=w519, type=w517, Variant=w518) -> (data=w516:T11)  [unwired: 1 out]
            }
          }
          n206 = Unbundle By Name(w506) -> ("Fs (Hz)"=w505:dbl, "atten (dB)"=w504:dbl, "Waveform"=w499:T12, "Freq Res (Hz)"=w503:dbl, "Order"=w500:i32, "Averages"=w502:i32, "seed"=w495:i64, "Window"=w494:T13)
          n207 = local write "Window"(w494) -> ()
          n208 = local write "Sample Rate (Hz)"(w505) -> ()
          n209 = local write "Attenuation (dB)"(w504) -> ()
          n210 = local write "Waveform"(w499) -> ()
          n211 = local write "Freq Step (Hz)"(w503) -> ()
          n212 = local write "Averages"(w502) -> ()
          n213 = local write "Seed"(w495) -> ()
          n214 = local write "Order"(w500) -> ()
          n215 = To Long Integer(number=w499) -> (32bit integer=w496:i32)
          n216 = Build Array (concatenate)("plot stim", "update window", w512) -> (w498:string[])
          n217 = local write "wftab"(w496) -> ()
        }
        frame "update window" {
          n218 = Unbundle By Name(w523) -> ("Window.Type"=w522:T14)
          n219 = Not Equal?(x=w522, y=HRTF-Window_Type."None") -> (x != y?=w520:bool)
          n220 = property on="Length (ms)" class="DigNum (strict)"("Visible"=w520) -> ()  [unwired: 2 in, 2 out]
          n221 = property on="Center (ms)" class="DigNum (strict)"("Visible"=w520) -> ()  [unwired: 2 in, 2 out]
        }
        frame "plot stim" {
          n222 = call "HRTF-Create Stimulus.vi"("Params"=w533) -> ("duration (ms)"=→"StimDur":dbl, "time"=→"Stimulus (time)":cluster{i32, "dx":dbl, "Y":dbl[]}, "autocorr"=→"StimAutocorr":cluster{dbl, "dx":dbl, "Y":dbl[]}, "mag"=→"StimMag":cluster{i32, "dx":dbl, "Y":dbl[]}, "phase"=→"StimPhase":cluster{i32, "dx":dbl, "Y":dbl[]})  [unwired: 9 in, 1 out]
          n223 = local write "Data Tab"(enum32{"Stimulus", "Response", "HRTFs"}."Stimulus" ("Data Tab")) -> ()
        }
        frame "do next" {
          n224 = invoke on="Config" class="HRTF Config (strict)" method="Select next.vi"() -> ("Select next.vi"=w538:i32)  [unwired: 3 in, 2 out]
          n225 = Unbundle By Name(w540) -> ("Azimuths"=w539:dbl[])
          n226 = Index Array(array=w539, index=w538) -> (element=w537:dbl)
          n227 = Bundle By Name(cluster=w544, "Azimuth"=w537, "iAzimuth"=w538) -> (w543:T16)
          n228 = case shown="0, Default" w538 {
            tunnel: w546 -> [w553 _]
            tunnel: w540 -> [w552 _]
            tunnel: w545 -> [w551 _]
            tunnel: w543 -> [w549 _]
            tunnel: [_ string[] ["end run"] ("String")] -> w542
            tunnel: [w547 u8 0] -> w541
            frame 0, Default {
              n229 = property on="Progress" class="Slide (strict)"() -> ("Value"=w548:u8)  [unwired: 2 in, 2 out]
              n230 = Bundle("Options"=w552, "Params"=w551, "State"=w549) -> (w550:T18)  [unwired: 1 in]
              n231 = Increment(x=w548) -> (x+1=w547:u8)
              n232 = Enqueue Element(queue=w553, element=w550) -> ()  [unwired: 2 in, 3 out]
            }
            frame -1 {
            }
          }
          n233 = property on="Progress" class="Slide (strict)"("Value"=w541) -> ()  [unwired: 2 in, 2 out]
        }
        frame "update" {
          n234 = Unbundle By Name(w558) -> ("Azimuths"=w557:dbl[])
          n235 = Unbundle By Name(w559) -> ("iAzimuth"=w560:i32)
          n236 = property on="Config" class="HRTF Config (strict)"("completed"=w560) -> ()  [unwired: 2 in, 2 out]
          n237 = call "HRTF-Enum Data Files.vi"("State"=w559, "Azimuths"=w557) -> ("file status"=w556:bool[][])  [unwired: 12 in, 1 out]
          n238 = property on="Config" class="HRTF Config (strict)"("file status"=w556) -> ()  [unwired: 2 in, 2 out]
        }
        frame "enum work" {
          n239 = Unbundle By Name(w570) -> ("Azimuths"=w569:dbl[])
          n240 = call "HRTF-Enum Data Files.vi"("State"=w568, "Azimuths"=w569) -> ("filestems"=w566:string[], "file status"=w567:bool[][])  [unwired: 12 in]
          n241 = Build Array (concatenate)("", w566) -> (w564:string[])
          n242 = property on="Config" class="HRTF Config (strict)"("file status"=w567) -> ()  [unwired: 2 in, 2 out]
          n243 = property on="RespFiles" class="Ring (strict)"("Strings []"=w564, "Value"=0) -> ()  [unwired: 2 in, 2 out]
        }
        frame "enum hrtfs" {
          n244 = Unbundle By Name(w580) -> ("Azimuths"=w579:dbl[])
          n245 = call "HRTF-Enum Data Files.vi"("State"=w578, "Azimuths"=w579, "HRTFs"=TRUE) -> ("filestems"=w577:string[])  [unwired: 11 in, 1 out]
          n246 = Build Array (concatenate)("", w577) -> (w574:string[])
          n247 = property on="HRTFFiles" class="Ring (strict)"("Strings []"=w574, "Value"=0) -> ()  [unwired: 2 in, 2 out]
        }
        frame "read work" {
          n248 = local read "RespFiles"() -> (w589:u16)
          n249 = property on="RespFiles" class="Ring (strict)"() -> ("Strings []"=w590:string[])  [unwired: 2 in, 2 out]
          n250 = Index Array(array=w590, index=w589) -> (element=w588:string)
          n251 = case shown="\"True\", Default" w588 {
            selector: w588 -> [_ w598]
            tunnel: w587 -> [_ w599]
            tunnel: [_ w597] -> w586
            tunnel: [_ w596] -> w585
            tunnel: [_ w595] -> w584
            tunnel: [_ w594] -> w583
            frame "" {
            }
            frame "True", Default {
              n252 = call "HRTF-Read Responses.vi"("State"=w599, "filestem"=w598) -> ("time"=w597:cluster{"offset":dbl, "dx":dbl, "Y":dbl[][]}, "crosscorr"=w596:cluster{"offset":dbl, "dx":dbl, "Y":dbl[][]}, "phase"=w594:cluster{"offset":dbl, "dx":dbl, "Y":dbl[][]}, "mag"=w595:cluster{"offset":dbl, "dx":dbl, "Y":dbl[][]})  [unwired: 9 in, 1 out]
            }
          }
          n253 = local write "RespTime"(w586) -> ()
          n254 = local write "RespCorr"(w585) -> ()
          n255 = local write "RespMag"(w584) -> ()
          n256 = local write "RespPhase"(w583) -> ()
        }
        frame "read hrtf" {
          n257 = property on="HRTFFiles" class="Ring (strict)"() -> ("RingText.Text"=w600:string)  [unwired: 2 in, 2 out]
          n258 = case shown="\"True\", Default" w600 {
            selector: w600 -> [_ w611]
            tunnel: w604 -> [_ w612]
            tunnel: [_ w610] -> w603
            tunnel: [_ w609] -> w602
            tunnel: [_ w608] -> w601
            frame "" {
            }
            frame "True", Default {
              n259 = call "HRTF-Read HRTFs.vi"("State"=w612, "filestem"=w611) -> ("IR"=w610:cluster{"offset":dbl, "dx":dbl, "Y":dbl[][]}, "phase"=w608:cluster{"offset":dbl, "dx":dbl, "Y":dbl[][]}, "mag"=w609:cluster{"offset":dbl, "dx":dbl, "Y":dbl[][]})  [unwired: 10 in, 1 out]
            }
          }
          "HRIR" <- w603
          "HRTFMag" <- w602
          "HRTFPhase" <- w601
        }
        frame "show hrtfs" {
          n260 = call "HRTF-Build Matfile Path.vi"("State"=w623) -> ("filestem"=w622:string)  [unwired: 13 in, 1 out]
          n261 = property on="HRTFFiles" class="Ring (strict)"() -> ("Strings []"=w617:string[])  [unwired: 2 in, 2 out]
          n262 = Array Size(array=w617) -> (size(s)=w616:i32)
          n263 = Search 1D Array(1D array=w617, element=w622) -> (index of element=w621:i32)  [unwired: 1 in]
          n264 = Greater?(x=w616, y=1) -> (0:w614:bool)
          n265 = Boolean To (0,1)(Boolean=w614) -> (0, 1=w613:i16)
          n266 = Max & Min(x=w621, y=w613) -> (max(x,y)=w620:i32)  [unwired: 1 out]
          n267 = local write "Data Tab"(enum32{"Stimulus", "Response", "HRTFs"}."HRTFs" ("Data Tab")) -> ()
          n268 = property on="HRTFFiles" class="Ring (strict)"("Value"=w620) -> ()  [unwired: 2 in, 2 out]
          n269 = Build Array (concatenate)(w625, "read hrtf") -> (w619:string[])
        }
        frame "end run" {
          n270 = property on="Config" class="HRTF Config (strict)"("highlight"=-1) -> ("selection"=w632:i32[])  [unwired: 2 in, 2 out]
          n271 = Array Size(array=w632) -> (size(s)=w631:i32)
          n272 = Greater Than 0?(x=w631) -> (x > 0?=w629:bool)
          n273 = call "Enable or Gray Out.vi"("Boolean"=w629) -> ("Disabled"=w628:T19)
          n274 = property on="Start" class="Bool"("Visible"=TRUE, "DisabledEnum"=w628) -> ()  [unwired: 2 in, 2 out]
          n275 = property on="RespFiles" class="Ring (strict)"("DisabledEnum"=T19."Enabled" ("Disabled")) -> ()  [unwired: 2 in, 2 out]
          n276 = property on="Status" class="Str"("Visible"=FALSE) -> ()  [unwired: 2 in, 2 out]
        }
        frame "enable start" {
          n277 = property on="Config" class="HRTF Config (strict)"() -> ("selection"=w640:i32[])  [unwired: 2 in, 2 out]
          n278 = Unbundle By Name(w644) -> ("Mic"=w642:i32, "Folder"=w648:path)
          n279 = Array Size(array=w640) -> (size(s)=w645:i32)
          n280 = Greater Than 0?(x=w642) -> (x > 0?=w641:bool)
          n281 = call "FileIO-File or Folder Exists.vi"("path"=w648) -> ("Exists?"=w649:bool)  [unwired: 7 in, 3 out]
          n282 = Greater Than 0?(x=w645) -> (x > 0?=w646:bool)
          n283 = Compound Arithmetic op=AND(w641, w649, w646) -> (w647:bool)
          n284 = call "Enable or Gray Out.vi"("Boolean"=w647) -> ("Disabled"=w643:T19)
          n285 = property on="Start" class="Bool"("DisabledEnum"=w643) -> ()  [unwired: 2 in, 2 out]
        }
        frame "compute" {
          w653 = T19."Enabled" ("Disabled")
          n286 = Unbundle By Name(w660) -> ("Fs (Hz)"=w659:dbl)
          n287 = control-ref of="Progress"() -> (w658:refnum<vi>)
          n288 = call "HRTF-Compute HRTFs.vi"("State"=w662, "Progress"=w658, "Window"="Window", "Desired Fs"=w659) -> ("error out"=w657:errorcluster)  [unwired: 11 in]
          n289 = call "Error Handler.vi"("error in (no error)"=w657) -> ("No Error"=w656:errorcluster)  [unwired: 13 in, 1 out]
          n290 = property on="Compute" class="Bool"(error in=w656, "DisabledEnum"=w653) -> ()  [unwired: 1 in, 2 out]
          n291 = property on="Start" class="Bool"("DisabledEnum"=w653) -> ()  [unwired: 2 in, 2 out]
          n292 = Build Array (concatenate)(w663, string[] ["show hrtfs", "enum hrtfs"] ("array")) -> (w655:string[])
        }
      }
      n293 = Empty Array?(array=w434) -> (empty?=w433:bool)
    }
  }
  n294 = while {
    tunnel: w16 -> [w668]
    tunnel: w13 -> [w665]
    stop <- w667 stop-if-true
    # "MEASUREMENT THREAD"
    n295 = Dequeue Element(queue=w668) -> (element=w666:T18, error out=w667:errorcluster)  [unwired: 2 in, 2 out]
    n296 = case shown="No Error" w667 {
      tunnel: w666 -> [w677 _]
      tunnel: w665 -> [w673 _]
      frame No Error {
        n297 = Unbundle By Name(w677) -> ("Options"=w676:T15, "Params"=w675:T11, "State"=w674:T16)
        n298 = while {
          shift-right: [w690] -> _
          shift-left: w676 -> [w693]
          shift-right: [w689] -> _
          shift-left: w675 -> [w692]
          shift-right: [w688] -> _
          shift-left: w674 -> [w691]
          tunnel: w673 -> [w686]
          shift-right: [w684] -> _
          shift-left: errorcluster {"status"=FALSE, "code"=0, "source"=""} ("error constant") -> [w685]
          shift-right: [w683] -> _
          shift-left: T23 {"StimSpec"=[], "Mic Sum"=[], "df (Hz)"=0.0, "dt (ms)"=0.0, "Navg"=0, "Nacq"=0, "pts/rep"=0, "reps/frame"=0, "Stimulus"=[]} ("Cal.Data") -> [w682]
          shift-right: [w680] -> _
          shift-left: T2 {"error"={"status"=FALSE, "code"=0, "source"=""}, "aborted"=FALSE} ("Value (Signaling)") -> [w681]
          shift-right: [w678] -> _
          shift-left: HRTF-State_Machine_Action."Wait" ("Action") -> [w679]
          stop <- w687 stop-if-true
          n299 = case shown="\"Multiplex\"" w679 {
            tunnel: w693 -> [w711 w744 w779 w804 w842 w852]
            tunnel: w692 -> [w712 w716 w778 w801 w831 w851]
            tunnel: w691 -> [w704 w728 w769 w793 w832 w850]
            tunnel: [w711 w744 w779 w804 w842 w852] -> w690
            tunnel: [w712 w716 w778 w801 w831 w851] -> w689
            tunnel: [w704 w728 w769 w793 w832 w850] -> w688
            tunnel: [_ _ _ _ _ TRUE] -> w687
            tunnel: w686 -> [w710 _ _ w799 _ _]
            tunnel: [w707 w739 w774 w796 HRTF-State_Machine_Action."End" ("Action") HRTF-State_Machine_Action."End" ("Action")] -> w678
            tunnel: w685 -> [w701 w742 w771 w803 w833 w846]
            tunnel: [w701 w741 w770 w794 w827 w846] -> w684
            tunnel: [w698 w729 w773 w788 w838 w845] -> w683
            tunnel: w682 -> [w698 _ w773 w800 w838 w845]
            tunnel: w681 -> [w697 w719 w772 w790 w839 w844]
            tunnel: [w696 w719 w772 w789 w839 w844] -> w680
            frame "Wait" {
              n300 = local write "Status"("Waiting..." ("Status")) -> ()
              n301 = Unbundle By Name(w711) -> ("Wait (s)"=w703:dbl)
              n302 = call "HRTF-Build Filename.vi"("State"=w704) -> ("filestem"=w694:string)  [unwired: 13 in, 1 out]
              n303 = control-ref of="RespFiles"() -> (w695:refnum<vi>)
              n304 = call "X1000.vi"("X"=w703) -> ("X/1000"=w702:dbl)
              n305 = call "HRTF-Add Filestem to Ring.vi"("Ring in"=w695, "filename"=w694) -> ()  [unwired: 14 in]
              n306 = local write "Data Tab"(enum32{"Stimulus", "Response", "HRTFs"}."Response" ("Data Tab")) -> ()
              n307 = Wait on Notification(notifier=w710, timeout in ms (-1)=w702) -> (timed out?=w705:bool)  [unwired: 2 in, 3 out]
              n308 = Not(x=w705) -> (.not. x?=w699:bool)
              n309 = Bundle By Name(cluster=w697, "aborted"=w699) -> (w696:T2)
              n310 = Select(t=HRTF-State_Machine_Action."End" ("Action"), s=w699, f=HRTF-State_Machine_Action."Init") -> (s? t:f=w707:T24)
            }
            frame "Init" {
              n311 = disable-structure shown="HARDWARE==TDT" {
                disable-tunnel: w742 -> [w752 w760]
                disable-tunnel: [w751 w753] -> w741
                disable-tunnel: [w750 w754] -> w736
                disable-tunnel: [w749 w756] -> w717
                disable-tunnel: w728 -> [w748 w758]
                disable-tunnel: w716 -> [w747 w759]
                disable-tunnel: [w746 w755] -> w720
                disable-tunnel: [w745 w757] -> w718
                frame condition #0 {
                  n312 = call "HRTF-Configure Hardware (NI).vi"("Params"=w747, "State"=w748, "error in (no error)"=w752) -> ("Stimulus"=w745:dbl[], "Sample Rate (Hz)"=w749:dbl, "pts/rep"=w746:i32, "reps/frame"=w750:i32, "error out"=w751:errorcluster)  [unwired: 8 in]
                }
                frame condition #1 (active) {
                  n313 = call "HRTF-Configure Hardware (TDT).vi"("Params"=w759, "State"=w758, "error in (no error)"=w760) -> ("Stimulus"=w757:dbl[], "Sample Rate (Hz)"=w756:dbl, "pts/rep"=w755:i32, "reps/frame"=w754:i32, "error out"=w753:errorcluster)  [unwired: 8 in]
                }
              }
              n314 = local write "Status"("Initializing..." ("Status")) -> ()
              n315 = Unbundle By Name(w716) -> ("Averages"=w725:i32)
              n316 = Unbundle By Name(w728) -> ("Mic"=w715:i32)
              n317 = Reverse 1D Array(array=w718) -> (reversed array=w724:dbl[])
              n318 = Not Equal?(x=w715, y=3) -> (x != y?=w714:bool)
              n319 = call-poly <vilib>:"FFT.vi"("X"=w724) -> ("FFT {X}"=w723:cdb[])  [unwired: 9 in, 1 out]
              n320 = Select(t=1, s=w714, f=2) -> (s? t:f=w721:i32)
              n321 = Build Array(w723, w723) -> (w722:cdb[][])
              n322 = Initialize Array(0.0 ("element"), w721, w720) -> (w730:dbl[][])
              n323 = Divide(x=1000.0, y=w717) -> (x/y=w735:dbl)
              n324 = Divide(x=w717, y=w720) -> (x/y=w733:dbl)
              n325 = Bundle By Name(cluster=T23 {"StimSpec"=[], "Mic Sum"=[], "df (Hz)"=0.0, "dt (ms)"=0.0, "Navg"=0, "Nacq"=0, "pts/rep"=0, "reps/frame"=0, "Stimulus"=[]} ("Cal.Data"), "StimSpec"=w722, "Stimulus"=w718, "pts/rep"=w720, "reps/frame"=w736, "dt (ms)"=w735, "df (Hz)"=w733, "Nacq"=0, "Mic Sum"=w730, "Navg"=w725) -> (w729:T23)
              n326 = Select(t=HRTF-State_Machine_Action."End" ("Action"), s=w741, f=HRTF-State_Machine_Action."Multiplex") -> (s? t:f=w739:T24)
            }
            frame "Multiplex" {
              w764 = T22 {"Output"={"Device"=enum."None", "Num"=0}, "Speaker"={"Channel"=0, "Primary mux"=0, "Secondary mux"=1}, "Right mic"=0, "Left mic"=1} ("TDT")
              n327 = call "Config File Path.vi"() -> ("Default config file name"=w765:path)  [unwired: 1 in]
              n328 = local write "Status"("Multiplexing..." ("Status")) -> ()
              n329 = Unbundle By Name(w769) -> ("iAzimuth"=w768:i32)
              n330 = call "Read Anything.vi"("Type of Anything"=w764, "Section Name (Name of \"Type of Anything\")"="TDT Config" ("Section Name (Name of \"Type of Anything\")"), "Path (dialog)"=w765) -> ("Anything"=w767:variant)  [unwired: 6 in, 2 out]
              n331 = Variant To Data(type=w764, Variant=w767) -> (data=w763:T22)  [unwired: 1 in, 1 out]
              n332 = Unbundle By Name(w763) -> ("Speaker.Primary mux"=w762:i32, "Speaker.Secondary mux"=w761:i32)
              n333 = disable-structure shown="HARDWARE==TDT" {
                disable-tunnel: w771 -> [w780 w783]
                disable-tunnel: [w780 w787] -> w770
                disable-tunnel: w768 -> [_ w786]
                disable-tunnel: w762 -> [_ w785]
                disable-tunnel: w761 -> [_ w784]
                frame condition #0 {
                  n334 = Wait (ms)(milliseconds to wait=u32 1000) -> ()  [unwired: 1 out]
                }
                frame condition #1 (active) {
                  n335 = call "TDT-Run Circuit.vi"("error in (no error)"=w783) -> ("error out"=w782:errorcluster)  [unwired: 14 in]
                  n336 = call "HRTF-Set Multiplexer (TDT).vi"("iAzimuth"=w786, "MUX 1"=w785, "MUX 2"=w784, "error in (no error)"=w782) -> ("error out"=w787:errorcluster)  [unwired: 11 in]
                }
              }
              n337 = Select(t=HRTF-State_Machine_Action."End" ("Action"), s=w770, f=HRTF-State_Machine_Action."Measure") -> (s? t:f=w774:T24)
            }
            frame "Measure" {
              n338 = call "SGDA-Start.vi"("error in (no error)"=w803) -> ("error out"=w802:errorcluster)  [unwired: 6 in]
              n339 = while {
                shift-right: [w811] -> w788
                shift-left: w800 -> [w825]
                shift-right: [w810] -> w794
                shift-left: w802 -> [w826]
                tunnel: w799 -> [w820]
                tunnel: [w817] -> w792
                tunnel: w793 -> [w809]
                i -> [w816]
                stop <- w818 stop-if-true
                n340 = call "SGDA-Read Data.vi"("error in (no error)"=w826) -> ("AI Waveforms"=w814:dbl[][], "error out"=w824:errorcluster)  [unwired: 13 in]
                n341 = Wait on Notification(notifier=w820, timeout in ms (-1)=0) -> (timed out?=w821:bool)  [unwired: 2 in, 3 out]
                n342 = Equal To 0?(x=w816) -> (x = 0?=w815:bool)
                n343 = Not(x=w821) -> (.not. x?=w817:bool)
                n344 = call "HRTF-Process Frame.vi"("Cal.Data In"=w825, "AI Waveforms"=w814, "First"=w815, "error in (no error)"=w824) -> ("Cal.Data Out"=w812:T23, "Status"=w823:string, "Finished"=w822:bool, "error out"=w813:errorcluster)  [unwired: 8 in]
                n345 = local write "Status"(w823) -> ()
                n346 = call "HRTF-Plot Response.vi"("Cal.Data in"=w812, "State"=w809, "error in (no error)"=w813) -> ("Cal.Data out"=w811:T23, "time"=→"RespTime":cluster{"offset":dbl, "dx":dbl, "Y":dbl[][]}, "crosscorr"=→"RespCorr":cluster{"offset":dbl, "dx":dbl, "Y":dbl[][]}, "phase"=→"RespPhase":cluster{"offset":dbl, "dx":dbl, "Y":dbl[][]}, "mag"=→"RespMag":cluster{"offset":dbl, "dx":dbl, "Y":dbl[][]}, "error out"=w810:errorcluster)  [unwired: 7 in]
                n347 = Compound Arithmetic op=OR(w810, w822, w817) -> (w818:bool)
              }
              n348 = Or(x=w794, y=w792) -> (x .or. y?=w795:bool)
              n349 = call "SGDA-Stop.vi"("error in (no error)"=w794) -> ("error out"=w791:errorcluster)  [unwired: 14 in]
              n350 = call <vilib>:"Clear Errors.vi"("error in (no error)"=w791) -> ()  [unwired: 5 in, 2 out]
              n351 = Bundle By Name(cluster=w790, "aborted"=w792) -> (w789:T2)
              n352 = Select(t=HRTF-State_Machine_Action."End" ("Action"), s=w795, f=HRTF-State_Machine_Action."Save") -> (s? t:f=w796:T24)
            }
            frame "Save" {
              n353 = Unbundle By Name(w838) -> ("Mic Sum"=w837:dbl[][], "Nacq"=w836:i32, "Stimulus"=w834:dbl[], "dt (ms)"=w830:dbl)
              n354 = local write "Status"("Saving..." ("Status")) -> ()
              n355 = Divide(x=w837, y=w836) -> (x/y=w835:dbl[][])
              n356 = call "Divide By 1000.vi"("X"=w830) -> ("X/1000"=w829:dbl)
              n357 = Reciprocal(x=w829) -> (1/x=w828:dbl)
              n358 = call "HRTF-Write Text File.vi"("Params"=w831, "State"=w832, "Data"=w835, "Stimulus"=w834, "error in (no error)"=w833, "Actual Fs"=w828) -> ("error out"=w827:errorcluster)  [unwired: 9 in]
            }
            frame "End", Default {
              n359 = local write "Status"("Done." ("Status")) -> ()
              n360 = Bundle By Name(cluster=w844, "error"=w846) -> (w847:T2)
              n361 = property on="Result" class="Clust (strict)"("Val(Sgnl)"=w847) -> ()  [unwired: 2 in, 2 out]
            }
          }
        }
      }
      frame Error {
      }
    }
  }
  n362 = disable-structure shown="RUN_TIME_ENGINE==True, Default" {
    disable-tunnel: w5 -> [w853 _]
    frame condition #0 {
      n363 = Quit LabVIEW(quit? (T)=w853) -> ()
    }
    frame condition #1 (active) {
    }
  }
